vi "2019-05-08_02.vi"() -> ()   [LabVIEW 2018]
panel:
  out "출력 클러스터 4":T1
  out "출력 클러스터 3":cluster{"Name":string, "Age":dbl}
  out "Age 3":dbl
  out "Name 3":string
  out "Age 2":dbl
  out "Address":string
  out "Student":bool
  out "Name 2":string
  in  "Applicant Cluster":T1
  out "출력 클러스터":cluster{"Name":string, "Age":dbl, "성별":bool}
  out "출력 클러스터 2":cluster{"Name":string, "Age":dbl, "성별":bool}
  in  "성별":bool
  in  "Age":dbl
  in  "Name":string
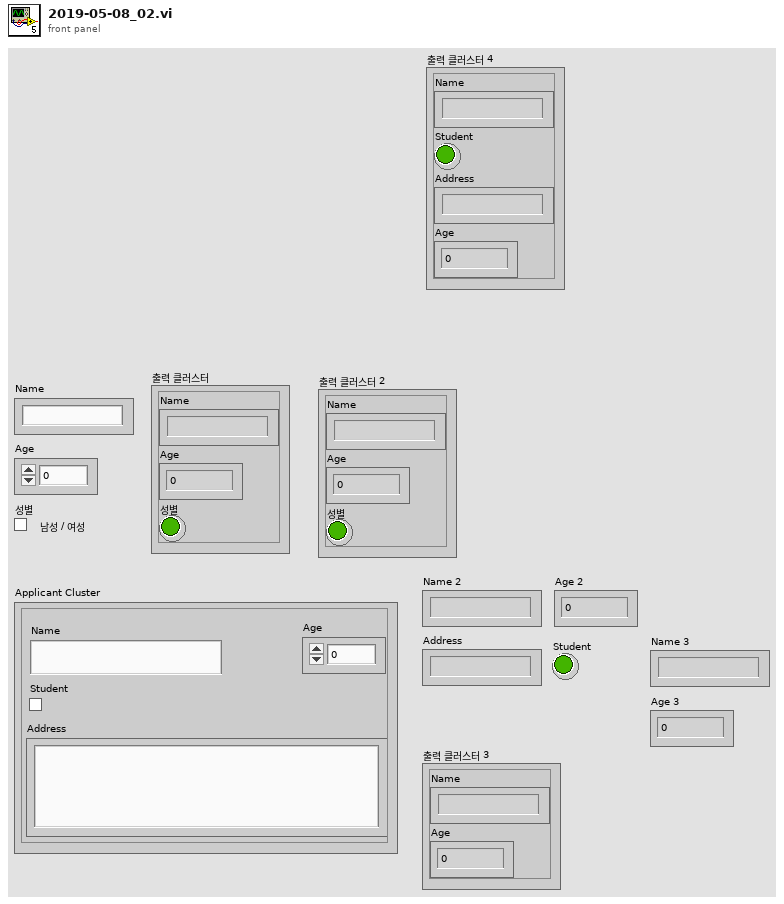
[diagram p1: front panel]
types:
  T1 = cluster{"Name":string, "Student":bool, "Address":string, "Age":dbl}
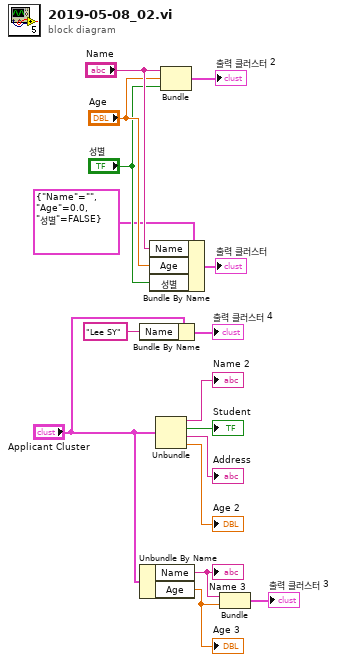
[diagram p0: block diagram]
diagram:
  n1 = Bundle By Name(cluster="Applicant Cluster", "Name"="Lee SY") -> (→"출력 클러스터 4":T1)
  n2 = Unbundle By Name("Applicant Cluster") -> ("Name"=w6:string, "Age"=w5:dbl)
  "Name 3" <- w6
  "Age 3" <- w5
  n3 = Bundle By Name(cluster=cluster{"Name":string, "Age":dbl, "성별":bool} {"Name"="", "Age"=0.0, "성별"=FALSE} ("출력 클러스터 3"), "Name"="Name", "Age"="Age", "성별"="성별") -> (→"출력 클러스터":cluster{"Name":string, "Age":dbl, "성별":bool})
  n4 = Unbundle("Applicant Cluster") -> ("Name"=→"Name 2":string, "Student"=→"Student":bool, "Address"=→"Address":string, "Age"=→"Age 2":dbl)
  n5 = Bundle("Name"="Name", "Age"="Age", "성별"="성별") -> (→"출력 클러스터 2":cluster{"Name":string, "Age":dbl, "성별":bool})  [unwired: 1 in]
  n6 = Bundle("Name"=w6, "Age"=w5) -> (→"출력 클러스터 3":cluster{"Name":string, "Age":dbl})  [unwired: 1 in]
